vi "QualityInit.vi"() -> (1 "DataSource Data":string[][](table), 2 "ColumnSetup":T1[](array[typedef]) {"MinWidth" min=2 step=1; "AutoSizeMode" items=["None"=1, "ColumnHeader"=2, "AllCellsExceptHeader"=4, "AllCells"=6, "DisplayedCellsExceptHeader"=8, "DisplayedCells"=10, "Fill"=16]; "FillWeight" min=1 max=100})   [LabVIEW 2020]
uses:
  <vilib>/DataGrid for LabVIEW/source/GridColumn/ColumnDefinition.ctl
  <vilib>/DataGrid for LabVIEW/source/GridColumn/ColumnType.ctl
  <vilib>/DataGrid for LabVIEW/source/GridColumn/GridColumn.lvclass
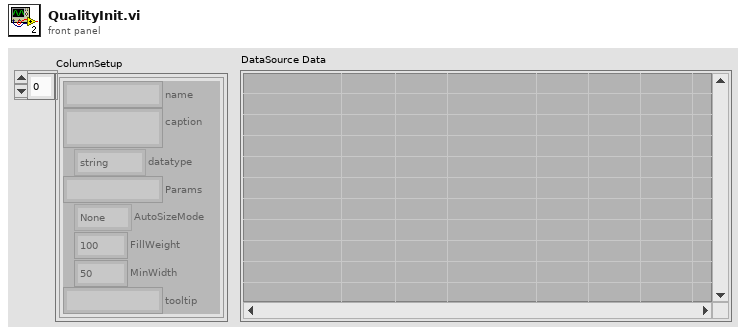
[diagram p1: front panel]
types:
  T1 = typedef "DataGrid.lvlib/GridColumn.lvclass/ColumnDefinition.ctl" = cluster{"name":string, "caption":string, "datatype":T2, "Params":string, "AutoSizeMode":i32, "FillWeight":sgl, "MinWidth":u32, "tooltip":string}
  T2 = typedef "DataGrid.lvlib/GridColumn.lvclass/ColumnType.ctl" = enum16{"string", "image", "check", "numeric", "timestamp", "button", "combo", "link"}
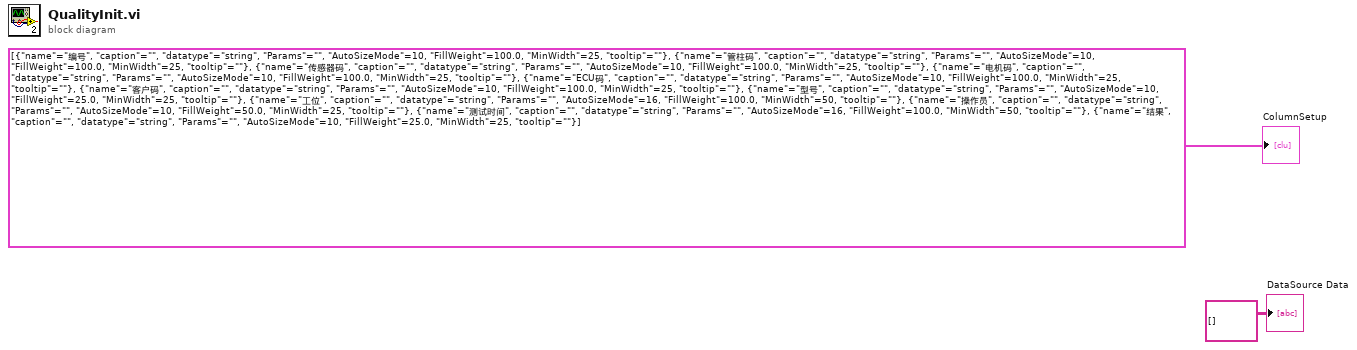
[diagram p0: block diagram]
diagram:
  "ColumnSetup" <- T1[] [{"name"="编号", "caption"="", "datatype"=enum."string", "Params"="", "AutoSizeMode"=10, "FillWeight"=100.0, "MinWidth"=25, "tooltip"=""}, {"name"="管柱码", "caption"="", "datatype"=enum."string", "Params"="", "AutoSizeMode"=10, "FillWeight"=100.0, "MinWidth"=25, "tooltip"=""}, {"name"="传感器码", "caption"="", "datatype"=enum."string", "Params"="", "AutoSizeMode"=10, "FillWeight"=100.0, "MinWidth"=25, "tooltip"=""}, {"name"="电机码", "caption"="", "datatype"=enum."string", "Params"="", "AutoSizeMode"=10, "FillWeight"=100.0, "MinWidth"=25, "tooltip"=""}, {"name"="ECU码", "caption"="", "datatype"=enum."string", "Params"="", "AutoSizeMode"=10, "FillWeight"=100.0, "MinWidth"=25, "tooltip"=""}, {"name"="客户码", "caption"="", "datatype"=enum."string", "Params"="", "AutoSizeMode"=10, "FillWeight"=100.0, "MinWidth"=25, "tooltip"=""}, {"name"="型号", "caption"="", "datatype"=enum."string", "Params"="", "AutoSizeMode"=10, "FillWeight"=25.0, "MinWidth"=25, "tooltip"=""}, {"name"="工位", "caption"="", "datatype"=enum."string", "Params"="", "AutoSizeMode"=16, "FillWeight"=100.0, "MinWidth"=50, "tooltip"=""}, {"name"="操作员", "caption"="", "datatype"=enum."string", "Params"="", "AutoSizeMode"=10, "FillWeight"=50.0, "MinWidth"=25, "tooltip"=""}, {"name"="测试时间", "caption"="", "datatype"=enum."string", "Params"="", "AutoSizeMode"=16, "FillWeight"=100.0, "MinWidth"=50, "tooltip"=""}, {"name"="结果", "caption"="", "datatype"=enum."string", "Params"="", "AutoSizeMode"=10, "FillWeight"=25.0, "MinWidth"=25, "tooltip"=""}] ("ColumnSetup")
  "DataSource Data" <- string[][] [] ("DataSource Data")
